vi "Motor Stop.vi"(8 "error in (no error)":errorcluster, 11 "Motor Controller in":refnum<class "Motor Controller.lvclass">) -> (0 "error out":errorcluster, 3 "Motor Controller out":refnum<class "Motor Controller.lvclass">)   [LabVIEW 2020, in "CTI-Peripheral.lvlib" / "Motor Controller.lvclass"]
uses:
  Motor Controller.lvclass
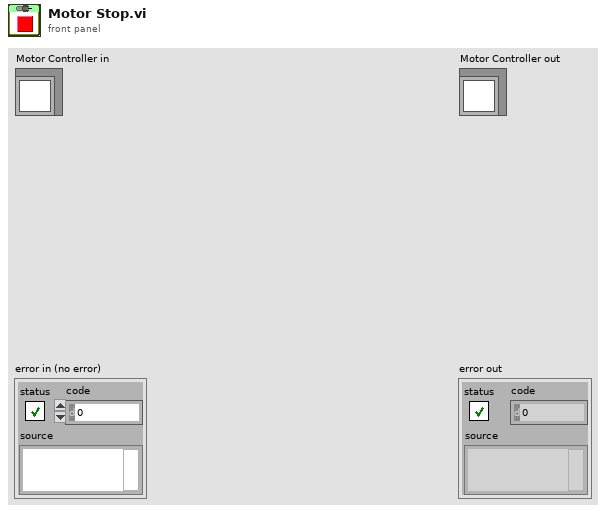
[diagram p1: front panel]
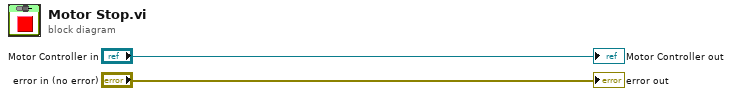
[diagram p0: block diagram]
diagram:
  "error out" <- "error in (no error)"
  "Motor Controller out" <- "Motor Controller in"
